vi "GetAPSxErrorString.vi"(8 "error in (no error)":errorcluster caption="错误输入（无错误）", 10 "ErrorCode":i32, 11 "PGIType":enum16{"APSX_PGI_TYPE_1", "APSX_PGI_TYPE_2"}(ring)=enum."APSX_PGI_TYPE_2") -> (0 "error out":errorcluster caption="错误输出", 3 "Message":string)   [LabVIEW 2020]
doc: "该模板用于创建子VI。"
uses:
  APSx.dll/APSx.dll
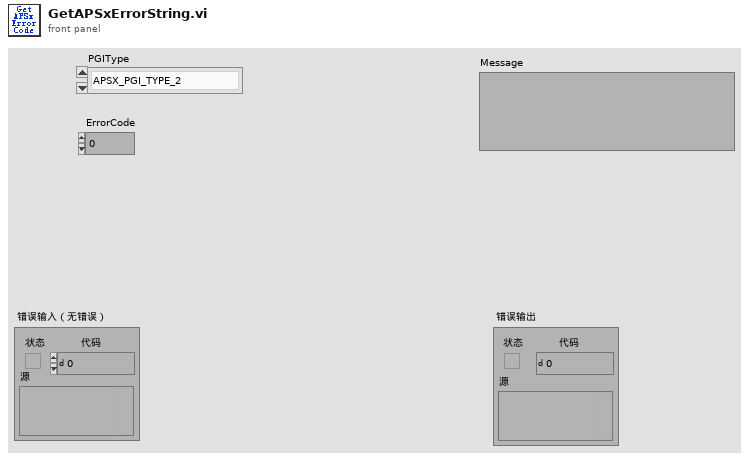
[diagram p1: front panel]
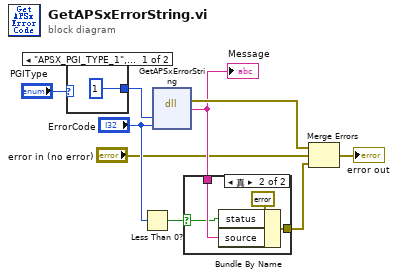
[diagram p0: block diagram]
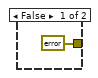
[diagram p2: hidden frame]
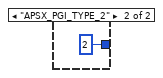
[diagram p3: hidden frame]
diagram:
  n1 = case shown="\"APSX_PGI_TYPE_1\", 默认" "PGIType" {
    tunnel: [1 2] -> w6
    frame "APSX_PGI_TYPE_1", Default {
    }
    frame "APSX_PGI_TYPE_2" {
    }
  }
  n2 = Less Than 0?(x="ErrorCode") -> (x < 0?=w2:bool)
  n3 = dll-call lib="PTH2iabs CUsersFengDesktop传感器对中台传感器对中台labviewSourcesAPSx.dllAPSx.dll" fn="GetAPSxErrorString"("PGIType"=w6, "ErrorCode"="ErrorCode") -> (error out=w9:errorcluster, "Message"=w3:string)  [unwired: 5 in, 1 out]
  "Message" <- w3
  n4 = case shown="真" w2 {
    selector: w2 -> [_ w13]
    tunnel: [errorcluster {"status"=FALSE, "code"=0, "source"=""} ("error in (no error)") w15] -> w4
    tunnel: w3 -> [_ w14]
    frame False {
    }
    frame True {
      n5 = Bundle By Name(cluster=errorcluster {"status"=FALSE, "code"=-9999, "source"=""} ("error in (no error)"), "status"=w13, "source"=w14) -> (w15:errorcluster)
    }
  }
  n6 = Merge Errors(w9, "error in (no error)", w4) -> (→"error out":errorcluster)
